vi "Write configuration.vi"(4 "predef positions":cluster{"pos_name":string, "pos_value":dbl}[][](array[cluster]), 6 "disabled flags":bool[](array[boolean]), 7 "email settings":T1, 8 "error in (no error)":errorcluster, 9 "setup ips":string[](array[string]), 10 "setup modes":string[](array[string]), 11 "ICS in":refnum<class "ICS.lvclass">) -> (0 "error out":errorcluster, 3 "ICS out":refnum<class "ICS.lvclass">)   [LabVIEW 2018, in "ICS.lvclass"]
uses:
  ICS.lvclass
  ICS.lvclass/ICS.ctl
  Motor/Motor.lvclass
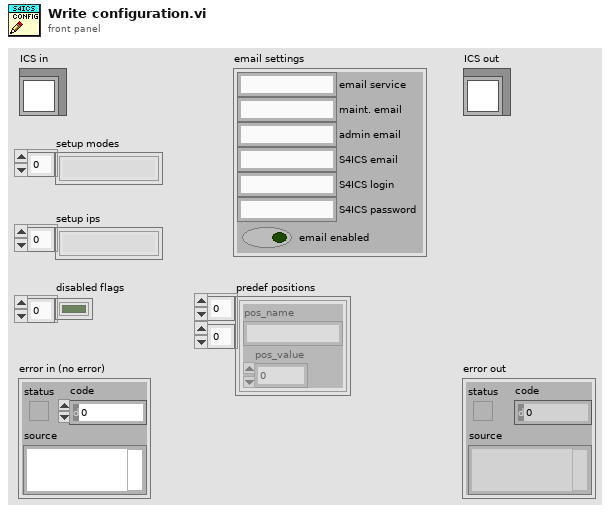
[diagram p1: front panel]
types:
  T1 = cluster{"email service":string, "maint. email":string, "admin email":string, "S4ICS email":string, "S4ICS login":string, "S4ICS password":string, "email enabled":bool}
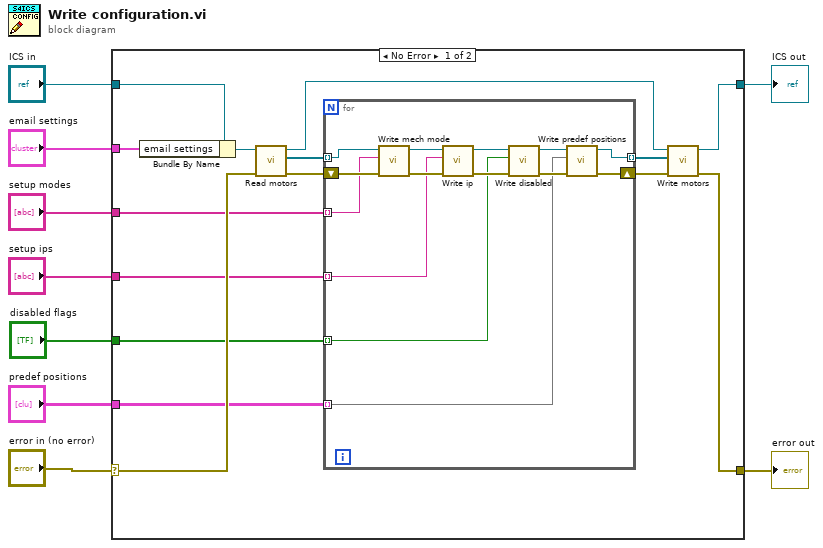
[diagram p0: block diagram]
diagram:
  n1 = case shown="No Error" "error in (no error)" {
    selector: "error in (no error)" -> [w21 w39]
    tunnel: [w12 w39] -> w8
    tunnel: [w13 w40] -> w6
    tunnel: "ICS in" -> [w23 w40]
    tunnel: "email settings" -> [w24 _]
    tunnel: "setup modes" -> [w18 _]
    tunnel: "setup ips" -> [w17 _]
    tunnel: "disabled flags" -> [w11 _]
    tunnel: "predef positions" -> [w10 _]
    frame No Error {
      n2 = Bundle By Name(cluster=w23, "email settings"=w24) -> (w22:refnum<class "ICS.lvclass">)
      n3 = call-dynamic "Read motors.vi"("error in (no error)"=w21, "ICS in"=w22) -> ("error out"=w20:errorcluster, "motors"=w19:refnum<class "Motor.lvclass">[], "ICS out"=w14:refnum<class "ICS.lvclass">)  [unwired: 7 in]
      n4 = for {
        shift-right: [w27] -> w16
        shift-left: w20 -> [w38]
        tunnel: w19 -> [w36] mode=indexing
        tunnel: w18 -> [w34] mode=indexing
        tunnel: w17 -> [w33] mode=indexing
        tunnel: [w26] -> w15 mode=indexing
        tunnel: w11 -> [w30] mode=indexing
        tunnel: w10 -> [w25] mode=indexing
        n5 = call-dynamic "Write mech mode.vi"("error in (no error)"=w38, "mech mode"=w34, "Motor in"=w36) -> ("error out"=w37:errorcluster, "Motor out"=w35:refnum<class "Motor.lvclass">)  [unwired: 7 in]
        n6 = call-dynamic "Write ip.vi"("error in (no error)"=w37, "ip"=w33, "Motor in"=w35) -> ("error out"=w32:errorcluster, "Motor out"=w31:refnum<class "Motor.lvclass">)  [unwired: 7 in]
        n7 = call-dynamic "Write disabled.vi"("error in (no error)"=w32, "disabled"=w30, "Motor in"=w31) -> ("error out"=w29:errorcluster, "Motor out"=w28:refnum<class "Motor.lvclass">)  [unwired: 7 in]
        n8 = call-dynamic "Write predef positions.vi"("error in (no error)"=w29, "predef positions"=w25, "Motor in"=w28) -> ("error out"=w27:errorcluster, "Motor out"=w26:refnum<class "Motor.lvclass">)  [unwired: 7 in]
      }
      n9 = call-dynamic "Write motors.vi"("error in (no error)"=w16, "motors"=w15, "ICS in"=w14) -> ("error out"=w12:errorcluster, "ICS out"=w13:refnum<class "ICS.lvclass">)  [unwired: 7 in]
    }
    frame Error {
    }
  }
  "error out" <- w8
  "ICS out" <- w6
